vi "FluxClose.vi"(1 "Error In":errorcluster, 2 "Master In":refnum<class "Modbus Master.lvclass">) -> (0 "Error Out":errorcluster)   [LabVIEW 2019]
uses:
  <vilib>/Modbus/master/Modbus Master.lvclass
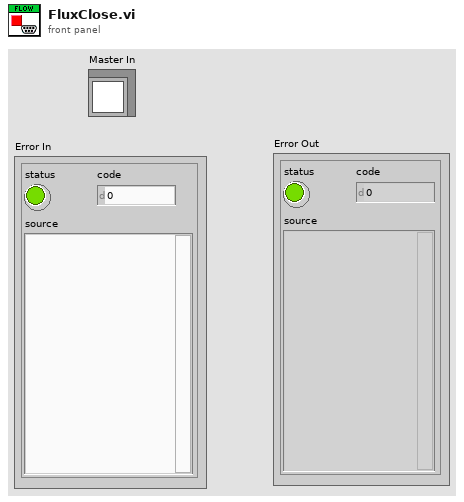
[diagram p1: front panel]
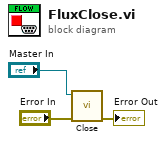
[diagram p0: block diagram]
diagram:
  n1 = call-dynamic "Close.vi"("error in (no error)"="Error In", "Modbus master in"="Master In") -> ("error out"=→"Error Out":errorcluster)  [unwired: 9 in]
